vi "Get to upper angle.vi"() -> ()   [LabVIEW 2013]
uses:
  InTake Global Data.vi
  Cannon/Cannon Global Data.vi
panel:
  out "finished":bool
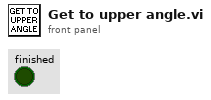
[diagram p1: front panel]
types:
  T1 = typedef "WPI_SolenoidValue.ctl" = enum16{"Off", "On", "Forward", "Reverse"}
  T2 = cluster{"MS":bool, "Shoot!":T1, "Angle":dbl, "Reset Gyro?":bool}
  T3 = cluster{"TakeBall":dbl, "UpperClaw":dbl, "LowerClaw":dbl, "MS":bool, "Angle":dbl}
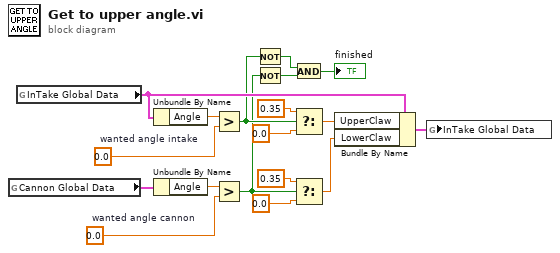
[diagram p0: block diagram]
diagram:
  w9 = 0.0  # wanted angle cannon
  w14 = 0.0  # wanted angle intake
  n1 = global read "Cannon Global Data.vi" "Cannon Global Data"() -> (w16:T2)
  n2 = global read "InTake Global Data.vi" "InTake Global Data"() -> (w17:T3)
  n3 = Unbundle By Name(w17) -> ("Angle"=w15:dbl)
  n4 = Unbundle By Name(w16) -> ("Angle"=w8:dbl)
  n5 = Greater?(x=w15, y=w14) -> (0:w5:bool)
  n6 = Greater?(x=w8, y=w9) -> (0:w4:bool)
  n7 = Not(x=w5) -> (.not. x?=w3:bool)
  n8 = Not(x=w4) -> (.not. x?=w2:bool)
  n9 = And(x=w3, y=w2) -> (x .and. y?=→"finished":bool)
  n10 = Select(t=0.35, s=w5, f=0.0) -> (s? t:f=w7:dbl)
  n11 = Select(t=0.35, s=w4, f=0.0) -> (s? t:f=w6:dbl)
  n12 = Bundle By Name(cluster=w17, "UpperClaw"=w7, "LowerClaw"=w6) -> (w18:T3)
  n13 = global write "InTake Global Data.vi" "InTake Global Data"(w18) -> ()
